vi "Get Size.vi"(8 "error in (no error)":errorcluster, 11 "Sequence of SBlocks in":refnum<class "Sequence of SBlocks.lvclass">) -> (0 "error out":errorcluster, 2 "size":i32, 3 "Sequence of SBlocks out":refnum<class "Sequence of SBlocks.lvclass">)   [LabVIEW 2020, in "TALOS.lvlib" / "Run Utilities.lvlib" / "Sequence of SBlocks.lvclass"]
uses:
  Sequence of SBlocks.lvclass
  Sequence of SBlocks.lvclass/Sequence of SBlocks.ctl
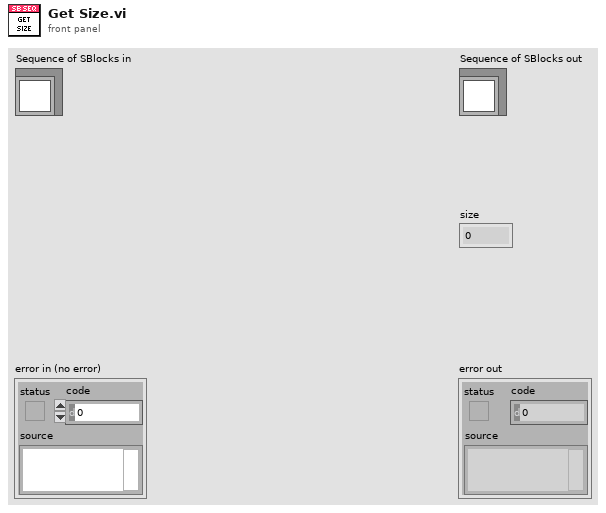
[diagram p1: front panel]
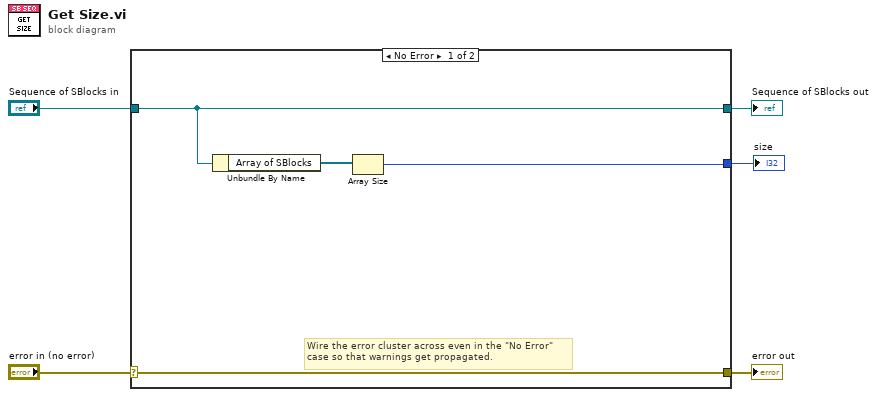
[diagram p0: block diagram]
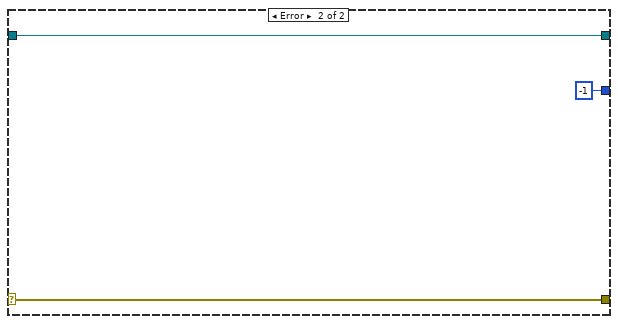
[diagram p2: hidden frame]
diagram:
  n1 = case shown="No Error" "error in (no error)" {
    selector: "error in (no error)" -> [w9 w12]
    tunnel: [w9 w12] -> w4
    tunnel: [w8 w11] -> w2
    tunnel: "Sequence of SBlocks in" -> [w8 w11]
    tunnel: [w6 -1] -> w1
    frame No Error {
      # "Wire the error cluster across even in the \"No Error\"\ncase so that warnings get propagated."
      n2 = Unbundle By Name(w8) -> ("Array of SBlocks"=w7:refnum<class "Schedule Block.lvclass">[])
      n3 = Array Size(array=w7) -> (size(s)=w6:i32)
    }
    frame Error {
    }
  }
  "error out" <- w4
  "Sequence of SBlocks out" <- w2
  "size" <- w1
